vi "getErrorDevice.vi"(8 "error in (no error)":errorcluster, 11 "AtomChipHWC in":refnum<class "AtomChipHWC.lvclass">) -> (0 "error out":errorcluster, 2 "Devices":string[](array[string]), 3 "AtomChipHWC out":refnum<class "AtomChipHWC.lvclass">)   [LabVIEW 2009, in "Hardware.lvlib" / "HWControllers.lvlib" / "AtomChipHWC.lvclass"]
uses:
  AtomChipHWC.lvclass
  AtomChipHWC.lvclass/AtomChipHWC.ctl
  HWController.lvclass
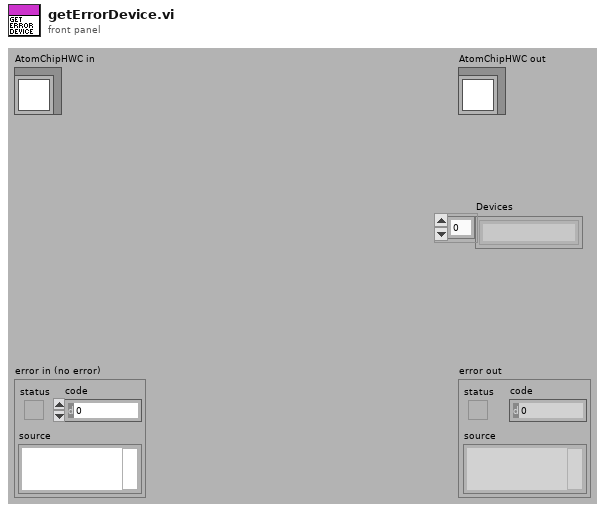
[diagram p1: front panel]
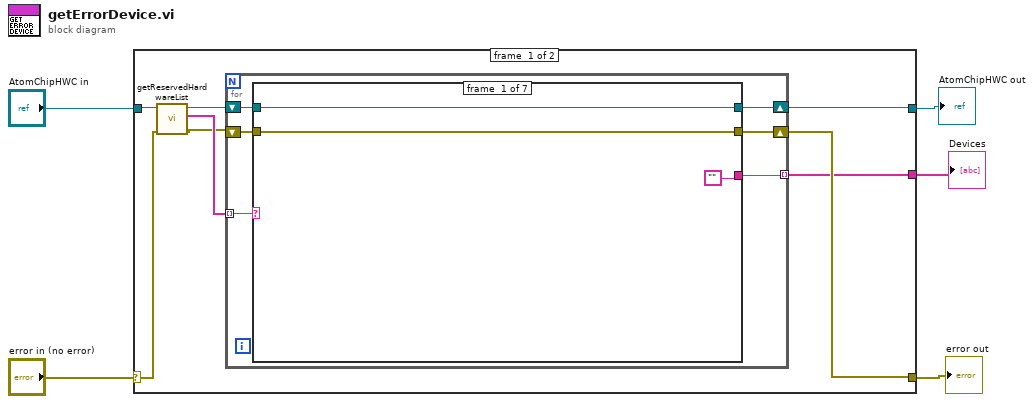
[diagram p0: block diagram]
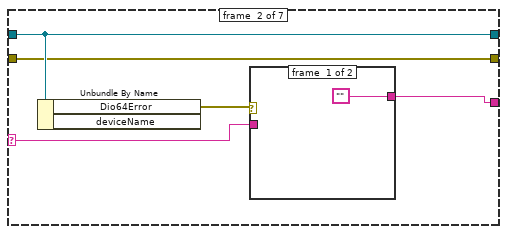
[diagram p2: hidden frame]
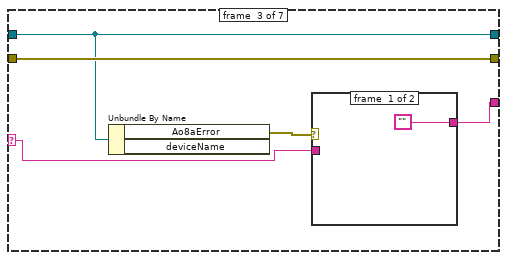
[diagram p4: hidden frame]
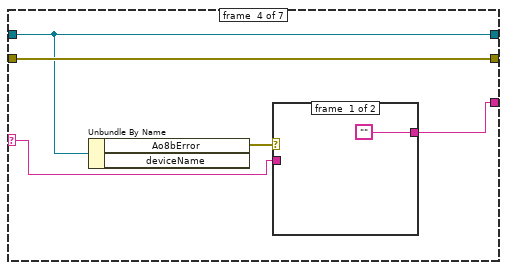
[diagram p6: hidden frame]
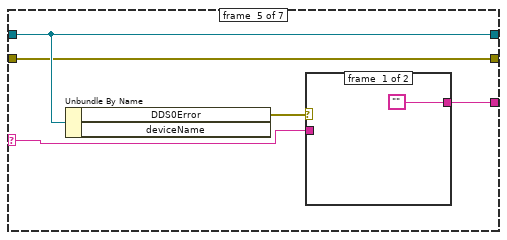
[diagram p8: hidden frame]
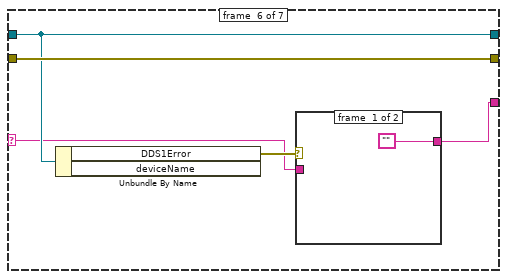
[diagram p10: hidden frame]
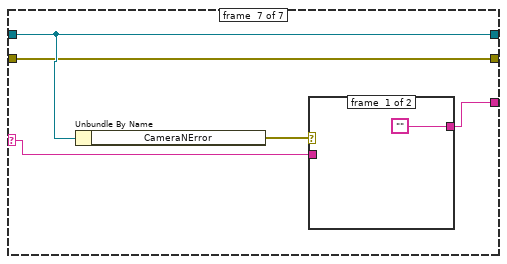
[diagram p12: hidden frame]
diagram:
  n1 = case shown="No Error" "error in (no error)" {
    selector: "error in (no error)" -> [w6 w66]
    tunnel: [w12 w66] -> w4
    tunnel: [w13 w65] -> w2
    tunnel: "AtomChipHWC in" -> [w10 w65]
    tunnel: [w11 _] -> w1
    frame #0 {
      n2 = call "getReservedHardwareList.vi"("error in (no error)"=w6, "HWController.lvclass in"=w10) -> ("error out"=w7:errorcluster, "reservedHardwareList"=w8:string[], "HWController.lvclass out"=w9:refnum<class "AtomChipHWC.lvclass">)  [unwired: 7 in]
      n3 = for {
        shift-right: [w18] -> w13
        shift-left: w9 -> [w19]
        tunnel: w8 -> [w16] mode=indexing
        shift-right: [w15] -> w12
        shift-left: w7 -> [w17]
        tunnel: [w14] -> w11 mode=indexing
        n4 = case shown="\"Dio64\"" w16 {
          selector: w16 -> [_ w23 w30 w37 w44 w51 w58]
          tunnel: w19 -> [w22 w27 w33 w40 w48 w52 w61]
          tunnel: [w22 w27 w33 w40 w48 w52 w61] -> w18
          tunnel: w17 -> [w21 w26 w34 w41 w47 w54 w60]
          tunnel: [w21 w26 w34 w41 w47 w54 w60] -> w15
          tunnel: ["" w24 w31 w38 w45 w53 w59] -> w14
          frame #0 {
          }
          frame #1 {
            n5 = Unbundle By Name(w27) -> ("Dio64Error"=w25:errorcluster)  [unwired: 1 out]
            n6 = case shown="Error" w25 {
              tunnel: ["" w29] -> w24
              tunnel: w23 -> [_ w29]
              frame #0 {
              }
              frame #1 {
              }
            }
          }
          frame #2 {
            n7 = Unbundle By Name(w33) -> ("Ao8aError"=w32:errorcluster)  [unwired: 1 out]
            n8 = case shown="Error" w32 {
              tunnel: ["" w36] -> w31
              tunnel: w30 -> [_ w36]
              frame #0 {
              }
              frame #1 {
              }
            }
          }
          frame #3 {
            n9 = Unbundle By Name(w40) -> ("Ao8bError"=w39:errorcluster)  [unwired: 1 out]
            n10 = case shown="Error" w39 {
              tunnel: ["" w43] -> w38
              tunnel: w37 -> [_ w43]
              frame #0 {
              }
              frame #1 {
              }
            }
          }
          frame #4 {
            n11 = Unbundle By Name(w48) -> ("DDS0Error"=w46:errorcluster)  [unwired: 1 out]
            n12 = case shown="No Error" w46 {
              tunnel: ["" w50] -> w45
              tunnel: w44 -> [_ w50]
              frame #0 {
              }
              frame #1 {
              }
            }
          }
          frame #5 {
            n13 = Unbundle By Name(w52) -> ("DDS1Error"=w55:errorcluster)  [unwired: 1 out]
            n14 = case shown="No Error" w55 {
              tunnel: ["" w57] -> w53
              tunnel: w51 -> [_ w57]
              frame #0 {
              }
              frame #1 {
              }
            }
          }
          frame #6 {
            n15 = Unbundle By Name(w61) -> ("CameraNError"=w62:errorcluster)
            n16 = case shown="Error" w62 {
              tunnel: ["" w64] -> w59
              tunnel: w58 -> [_ w64]
              frame #0 {
              }
              frame #1 {
              }
            }
          }
        }
      }
    }
    frame #1 {
    }
  }
  "error out" <- w4
  "AtomChipHWC out" <- w2
  "Devices" <- w1
